vi "Append Log List.vi"(8 "error in (no error)":errorcluster, 10 "log list":string[](array[string]), 11 "Normal Log in":refnum<class "Normal Log.lvclass">) -> (0 "error out":errorcluster, 3 "Normal Log out":refnum<class "Normal Log.lvclass">)   [LabVIEW 2020, in "Normal Log.lvlib" / "Normal Log.lvclass"]
uses:
  Normal Log.lvclass
  <vilib>/Utility/miscctls.llb/LVRowAndColumnUnsignedTypeDef.ctl
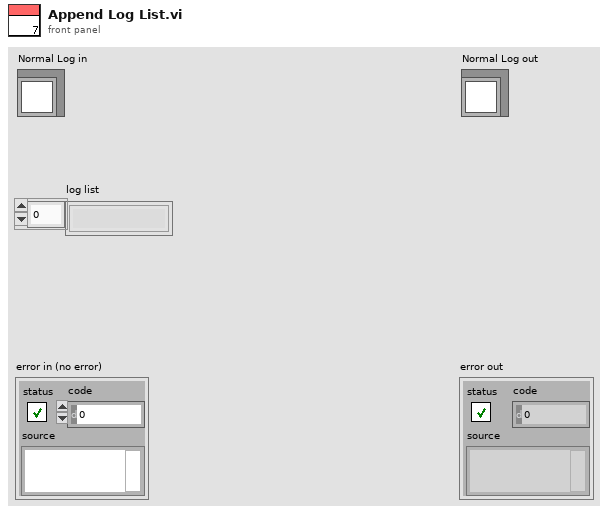
[diagram p1: front panel]
types:
  T1 = typedef "LVRowAndColumnUnsignedTypeDef.ctl" = cluster{"Row":u32, "Column":u32}
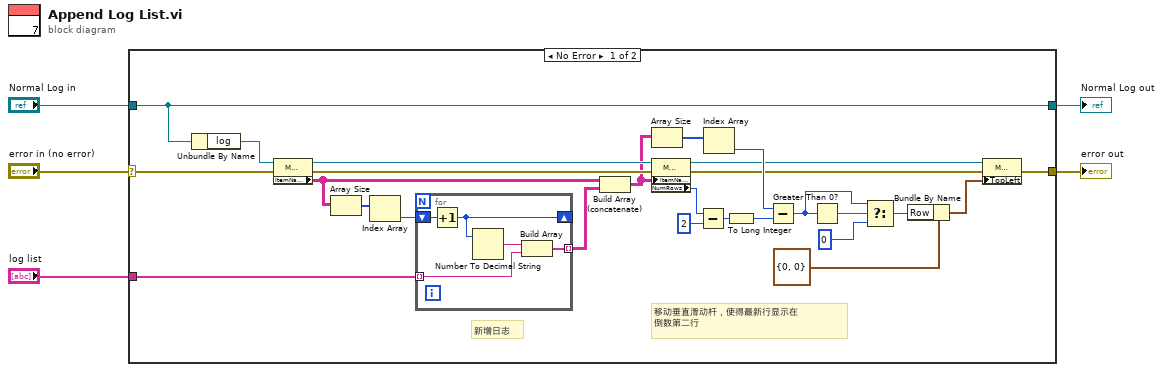
[diagram p0: block diagram]
diagram:
  n1 = case shown="No Error" "error in (no error)" {
    selector: "error in (no error)" -> [w24 w38]
    tunnel: "log list" -> [w22 _]
    tunnel: "Normal Log in" -> [w23 w37]
    tunnel: [w10 w38] -> w2
    tunnel: [w23 w37] -> w1
    frame No Error {
      # "移动垂直滑动杆，使得最新行显示在\n倒数第二行"
      # "新增日志"
      n2 = Unbundle By Name(w23) -> ("log"=w25:refnum<vi>)
      n3 = property class="MCListbox (strict)"(reference=w25, error in=w24) -> (reference out=w27:refnum<vi>, error out=w26:errorcluster, "ItemNames"=w28:string[][])
      n4 = Array Size(array=w28) -> (size(s)=w29:i32[])
      n5 = Index Array(array=w29) -> (element=w30:i32)  [unwired: 1 in]
      n6 = for {
        tunnel: w22 -> [w33] mode=indexing
        shift-right: [w35] -> _
        shift-left: w30 -> [w36]
        tunnel: [w32] -> w31 mode=indexing
        n7 = Increment(x=w36) -> (x+1=w35:i32)
        n8 = Number To Decimal String(number=w35) -> (decimal integer string=w34:string)  [unwired: 1 in]
        n9 = Build Array(w34, w33) -> (w32:string[])
      }
      n10 = Build Array (concatenate)(w28, w31) -> (w20:string[][])
      n11 = Array Size(array=w20) -> (size(s)=w21:i32[])
      n12 = property class="MCListbox (strict)"(reference=w27, error in=w26, "ItemNames"=w20) -> (reference out=w13:refnum<vi>, error out=w14:errorcluster, "NumRows"=w17:u32)
      n13 = Subtract(x=w17, y=u32 2) -> (x-y=w18:u32)
      n14 = Index Array(array=w21) -> (element=w15:i32)  [unwired: 1 in]
      n15 = To Long Integer(number=w18) -> (32bit integer=w16:i32)
      n16 = Subtract(x=w15, y=w16) -> (x-y=w8:i32)
      n17 = Greater Than 0?(x=w8) -> (x > 0?=w9:bool)
      n18 = Select(t=w8, s=w9, f=0 ("y")) -> (s? t:f=w6:i32)
      n19 = Bundle By Name(cluster=T1 {"Row"=0, "Column"=0} ("Top Left Visible Cell"), "Row"=w6) -> (w12:T1)
      n20 = property class="MCListbox (strict)"(reference=w13, error in=w14, "TopLeft"=w12) -> (error out=w10:errorcluster)  [unwired: 1 out]
    }
    frame Error {
    }
  }
  "error out" <- w2
  "Normal Log out" <- w1
